vi "onCreatePublishPacket.vi"(4 "RETAIN":bool, 5 "PUBLISH type":refnum<class "PUBLISH.lvclass">, 6 "QoS":T1, 7 "DUP (Re-delivery attempt)":bool, 8 "error in (no error)":errorcluster, 9 "Packet ID (empty: generate new)":u16 format="%04x", 10 "Payload":u8[](array[numeric]) format="%08b", 11 "Topic Name":string) -> (0 "error out":errorcluster, 1 "Packet ID":u16 format="%04x", 2 "Bytes Stream":u8[](array[numeric]) format="%08b", 3 "PUBLISH":refnum<class "PUBLISH.lvclass">)   [LabVIEW 2013, in "MQTT_Control_Packets.lvlib" / "PUBLISH.lvclass"]
uses:
  PUBLISH.lvclass
  ControlPacket/QualityOfService -- enum.ctl
  ControlPacket/ControlPacket.lvclass/ControlPacket.ctl
  ControlPacket/ControlPacket.lvclass
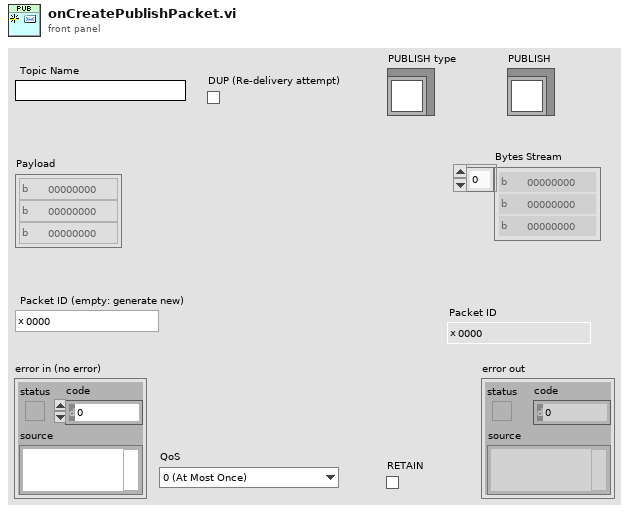
[diagram p1: front panel]
types:
  T1 = typedef "MQTT_Control_Packets.lvlib/ControlPacket.lvclass/QualityOfService -- enum.ctl" = enum16{"0 (At Most Once)", "1 (At Least Once)", "2 (Exactly Once)"}
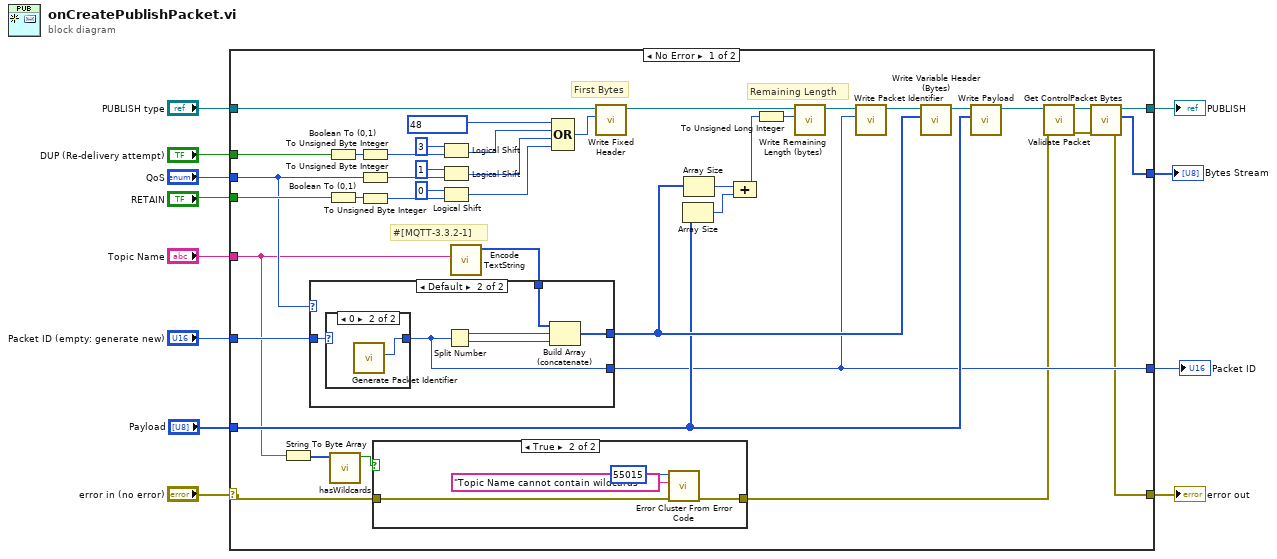
[diagram p0: block diagram]
diagram:
  n1 = case shown="No Error" "error in (no error)" {
    selector: "error in (no error)" -> [w19 w69]
    tunnel: [w14 w69] -> w11
    tunnel: [w16 w68] -> w9
    tunnel: "PUBLISH type" -> [w39 w68]
    tunnel: "DUP (Re-delivery attempt)" -> [w40 _]
    tunnel: "RETAIN" -> [w53 _]
    tunnel: "QoS" -> [w23 _]
    tunnel: "Topic Name" -> [w21 _]
    tunnel: "Packet ID (empty: generate new)" -> [w26 _]
    tunnel: "Payload" -> [w32 _]
    tunnel: [w25 _] -> w2
    tunnel: [w13 _] -> w1
    frame No Error {
      # "#[MQTT-3.3.2-1]"
      # "Remaining Length"
      # "First Bytes"
      n2 = String To Byte Array(string=w21) -> (unsigned byte array=w22:u8[])
      n3 = Boolean To (0,1)(Boolean=w40) -> (0, 1=w49:i16)
      n4 = Boolean To (0,1)(Boolean=w53) -> (0, 1=w48:i16)
      n5 = call "hasWildcards.vi"("Topic Name (Bytes Array)"=w22) -> ("has Wildcards"=w20:bool)  [unwired: 10 in]
      n6 = To Unsigned Byte Integer(number=w49) -> (unsigned 8bit integer=w50:u8)
      n7 = To Unsigned Byte Integer(number=w23) -> (unsigned 8bit integer=w47:u8)
      n8 = To Unsigned Byte Integer(number=w48) -> (unsigned 8bit integer=w46:u8)
      n9 = case shown="True" w20 {
        tunnel: w19 -> [w54 w57]
        tunnel: [w54 w58] -> w18
        frame False {
        }
        frame True {
          n10 = call <vilib>:"Error Cluster From Error Code.vi"("error in (no error)"=w57, "error message (\"\")"="Topic Name cannot contain wildcards" ("error message (\"\")"), "error code (0)"=55015) -> ("error out"=w58:errorcluster)  [unwired: 6 in]
        }
      }
      n11 = Logical Shift(y=i16 3, x=w50) -> (x << y=w51:u8)
      n12 = Logical Shift(y=i16 1, x=w47) -> (x << y=w45:u8)
      n13 = Logical Shift(y=i16 0, x=w46) -> (x << y=w44:u8)
      n14 = call "Encode TextString.vi"("Text String"=w21) -> ("Length-Prefixed Field"=w34:u8[])  [unwired: 10 in]
      n15 = case shown="Default" w23 {
        tunnel: w34 -> [w59 w65]
        tunnel: [w59 w62] -> w33
        tunnel: w26 -> [_ w61]
        tunnel: [_ w60] -> w25
        frame "0 (At Most Once)" {
          # "#[MQTT-2.3.1-5]"
        }
        frame Default {
          n16 = case shown="0" w61 {
            selector: w61 -> [w66 _]
            tunnel: [w66 w67] -> w60
            frame Default {
            }
            frame 0 {
              n17 = call "Generate Packet Identifier.vi"() -> ("Packet Identifier"=w67:u16)  [unwired: 11 in]
            }
          }
          n18 = Split Number(x=w60) -> (hi(x)=w64:u8, lo(x)=w63:u8)
          n19 = Build Array (concatenate)(w65, w64, w63) -> (w62:u8[])
        }
      }
      n20 = Compound Arithmetic op=OR(u8 48, w51, w45, w44) -> (w38:u8)
      n21 = call "Write Fixed Header.vi"("Fixed Header"=w38, "ControlPacket in"=w39) -> ("ControlPacket out"=w36:refnum<class "PUBLISH.lvclass">)  [unwired: 9 in]
      n22 = Array Size(array=w32) -> (size(s)=w30:i32)
      n23 = Array Size(array=w33) -> (size(s)=w31:i32)
      n24 = Compound Arithmetic op=ADD(w31, w30) -> (w29:i32)
      n25 = To Unsigned Long Integer(number=w29) -> (unsigned 32bit integer=w37:u32)
      n26 = call "Write Remaining Length (bytes).vi"("Remaining Length (bytes)"=w37, "ControlPacket in"=w36) -> ("ControlPacket out"=w28:refnum<class "PUBLISH.lvclass">)  [unwired: 9 in]
      n27 = call "Write Packet Identifier.vi"("Packet Identifier"=w25, "ControlPacket in"=w28) -> ("ControlPacket out"=w27:refnum<class "PUBLISH.lvclass">)  [unwired: 9 in]
      n28 = call "Write Variable Header (Bytes).vi"("Variable Header (Bytes)"=w33, "ControlPacket in"=w27) -> ("ControlPacket out"=w35:refnum<class "PUBLISH.lvclass">)  [unwired: 9 in]
      n29 = call "Write Payload.vi"("Payload"=w32, "ControlPacket in"=w35) -> ("ControlPacket out"=w24:refnum<class "PUBLISH.lvclass">)  [unwired: 9 in]
      n30 = call "Validate Packet.vi"("error in (no error)"=w18, "ControlPacket in"=w24) -> ("error out"=w15:errorcluster, "ControlPacket out"=w17:refnum<class "PUBLISH.lvclass">)  [unwired: 8 in]
      n31 = call "Get ControlPacket Bytes.vi"("error in (no error)"=w15, "ControlPacket"=w17) -> ("error out"=w14:errorcluster, "Bytes Stream"=w13:u8[], "ControlPacket dup"=w16:refnum<class "PUBLISH.lvclass">)  [unwired: 6 in, 1 out]
    }
    frame Error {
    }
  }
  "error out" <- w11
  "PUBLISH" <- w9
  "Packet ID" <- w2
  "Bytes Stream" <- w1
